vi "xps_panel_DO_dither_stage.vi"(8 "error in (no error)":errorcluster, 11 "newport_xps_panel in":refnum<class "newport_xps_panel.lvclass">) -> (0 "error out":errorcluster, 3 "newport_xps_panel out":refnum<class "newport_xps_panel.lvclass">)   [LabVIEW 2015, in "newport_xps_panel.lvclass"]
uses:
  newport_xps_panel.lvclass
  newport_xps/newport_xps.lvclass
  UI/panel_class/panel.lvclass
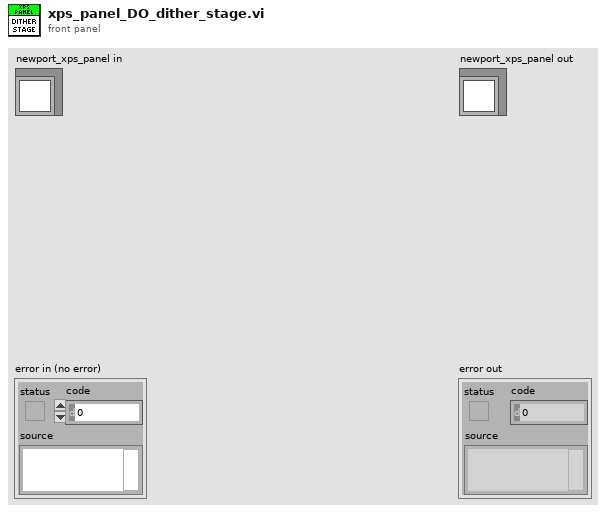
[diagram p1: front panel]
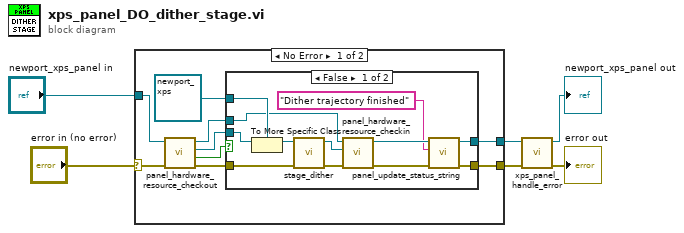
[diagram p0: block diagram]
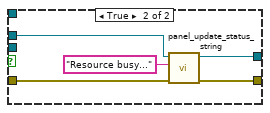
[diagram p2: hidden frame]
diagram:
  n1 = case shown="No Error" "error in (no error)" {
    selector: "error in (no error)" -> [w15 w34]
    tunnel: [w9 w34] -> w4
    tunnel: [w8 w33] -> w1
    tunnel: "newport_xps_panel in" -> [w14 w33]
    frame No Error {
      n2 = call "panel_hardware_resource_checkout.vi"("error in (no error)"=w15, "panel in"=w14) -> ("error out"=w10:errorcluster, "timed out?"=w13:bool, "hardware.lvclass"=w11:refnum<class "hardware.lvclass">, "panel out"=w12:refnum<class "newport_xps_panel.lvclass">)  [unwired: 6 in]
      n3 = case shown="False" w13 {
        tunnel: w12 -> [w17 w29]
        tunnel: w11 -> [w27 _]
        tunnel: w10 -> [w19 w32]
        tunnel: [w23 w31] -> w9
        tunnel: [w22 w28] -> w8
        tunnel: refnum<class "newport_xps.lvclass"> refnum ("newport_xps in") -> [w26 _]
        frame False {
          n4 = To More Specific Class(target class=w26, reference=w27) -> (specific class reference=w21:refnum<class "newport_xps.lvclass">)  [unwired: 1 in, 1 out]
          n5 = call-dynamic "stage_dither.vi"("error in (no error)"=w19, "newport_xps in"=w21) -> ("error out"=w18:errorcluster, "newport_xps out"=w20:refnum<class "newport_xps.lvclass">)  [unwired: 8 in]
          n6 = call "panel_hardware_resource_checkin.vi"("error in (no error)"=w18, "hardware.lvclass"=w20, "panel in"=w17) -> ("error out"=w25:errorcluster, "panel out"=w24:refnum<class "newport_xps_panel.lvclass">)  [unwired: 7 in]
          n7 = call-dynamic "panel_update_status_string.vi"("error in (no error)"=w25, "String"="Dither trajectory finished", "newport_xps_panel in"=w24) -> ("error out"=w23:errorcluster, "newport_xps_panel out"=w22:refnum<class "newport_xps_panel.lvclass">)  [unwired: 7 in]
        }
        frame True {
          n8 = call-dynamic "panel_update_status_string.vi"("error in (no error)"=w32, "String"="Resource busy...", "newport_xps_panel in"=w29) -> ("error out"=w31:errorcluster, "newport_xps_panel out"=w28:refnum<class "newport_xps_panel.lvclass">)  [unwired: 7 in]
        }
      }
    }
    frame Error {
    }
  }
  n9 = call "xps_panel_handle_error.vi"("error in (no error)"=w4, "newport_xps_panel in"=w1) -> ("error out"=→"error out":errorcluster, "newport_xps_panel out"=→"newport_xps_panel out":refnum<class "newport_xps_panel.lvclass">)  [unwired: 8 in]
